vi "MoveElbow.vi"(8 "error in (no error)":errorcluster caption="Fehler (Eingang, kein Fehler)", 9 "Speed":i16=300, 10 "Elbow":dbl, 11 "Moveo Eingang":refnum<class "Moveo.lvclass">) -> (0 "error out":errorcluster caption="Fehler (Ausgang)", 3 "Moveo Ausgang":refnum<class "Moveo.lvclass">)   [LabVIEW 2019, in "Moveo.lvclass"]
uses:
  Moveo.lvclass
  Moveo.lvclass/Moveo.ctl
  MoveoSerialClass/MoveoSerial.lvclass
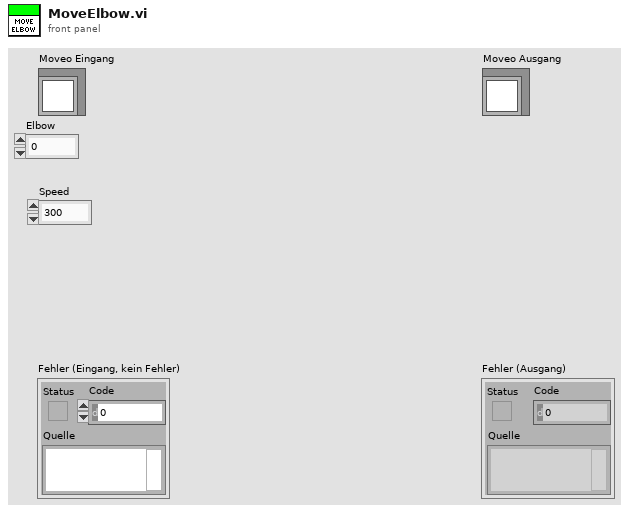
[diagram p1: front panel]
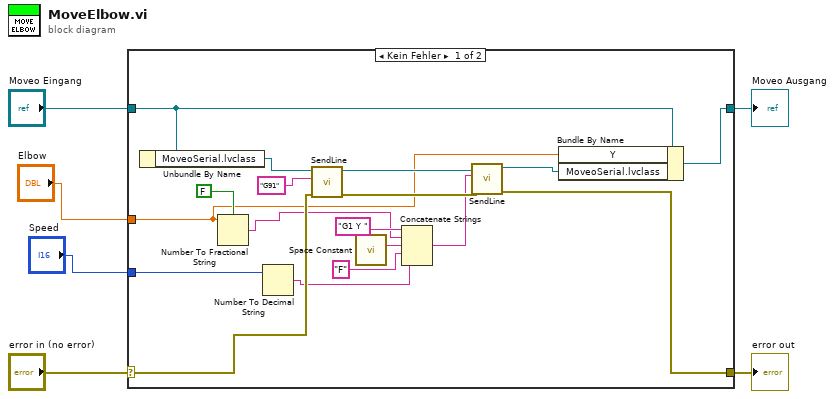
[diagram p0: block diagram]
diagram:
  n1 = case shown="Kein Fehler" "error in (no error)" {
    selector: "error in (no error)" -> [w20 w26]
    tunnel: [w9 w26] -> w5
    tunnel: [w7 w25] -> w3
    tunnel: "Moveo Eingang" -> [w11 w25]
    tunnel: "Elbow" -> [w8 _]
    tunnel: "Speed" -> [w22 _]
    frame No Error {
      n2 = Unbundle By Name(w11) -> ("MoveoSerial.lvclass"=w24:refnum<class "MoveoSerial.lvclass">)
      n3 = Number To Fractional String(use system decimal point (T)=FALSE ("Systemdezimalzeichen verwenden (T)"), number=w8) -> (F-format string=w16:string)  [unwired: 2 in]
      n4 = Number To Decimal String(number=w22) -> (decimal integer string=w15:string)  [unwired: 1 in]
      n5 = call-dynamic "SendLine.vi"("error in (no error)"=w20, "SendString"="G91", "MoveoSerial Eingang"=w24) -> ("error out"=w13:errorcluster, "MoveoSerial Ausgang"=w14:refnum<class "MoveoSerial.lvclass">)  [unwired: 7 in]
      n6 = call <vilib>:"Space Constant.vi"() -> ("String"=w18:string)
      n7 = Concatenate Strings("G1 Y ", w16, w18, "F", w15) -> (w12:string)
      n8 = call-dynamic "SendLine.vi"("error in (no error)"=w13, "SendString"=w12, "MoveoSerial Eingang"=w14) -> ("error out"=w9:errorcluster, "MoveoSerial Ausgang"=w10:refnum<class "MoveoSerial.lvclass">)  [unwired: 7 in]
      n9 = Bundle By Name(cluster=w11, "Y"=w8, "MoveoSerial.lvclass"=w10) -> (w7:refnum<class "Moveo.lvclass">)
    }
    frame Error {
    }
  }
  "error out" <- w5
  "Moveo Ausgang" <- w3
